vi "GUI.DisableState.Set.vi"(7 "Enable?":bool=TRUE, 8 "error in (no error)":errorcluster, 11 "State Variables in":T1) -> (0 "error out":errorcluster, 3 "State Variables out":T1)   [LabVIEW 2025, in "XNET Bus Monitor Client.lvlib"]
uses:
  XNET Bus Monitor Client.lvlib
  Types/GUI.StateVariables.ctl
  Types/StreamEngine.CmdQueueData.ctl
  Types/StreamEngine.CmdQueueData.Cmd.ctl
  Types/StreamEngine.QueueRefs.ctl
  Types/GUI.Controls.Refs.ctl
  <vilib>/gRPC/LabVIEW gRPC Library/Shared/grpcId.ctl
  <vilib>/gRPC/LabVIEW gRPC Library/grpc-lvsupport-release.lvlib
  xnet_can_bus_monitor_api_client/RPC Messages/ni_xnet_can_bm_api_DirectionFilter.ctl
  xnet_can_bus_monitor_api_client/xnet_can_bus_monitor_api_client.lvlib
  xnet_can_bus_monitor_api_client/RPC Messages/ni_xnet_can_bm_api_FrameFilter.ctl
  Types/gRPC.ConnectionInfo.ctl
  Types/SubProcessEngine.CmdQueueData.ctl
  Types/SubProcessEngine.CmdQueueData.Cmd.ctl
  Types/SubProcessEngine.QueueRefs.ctl
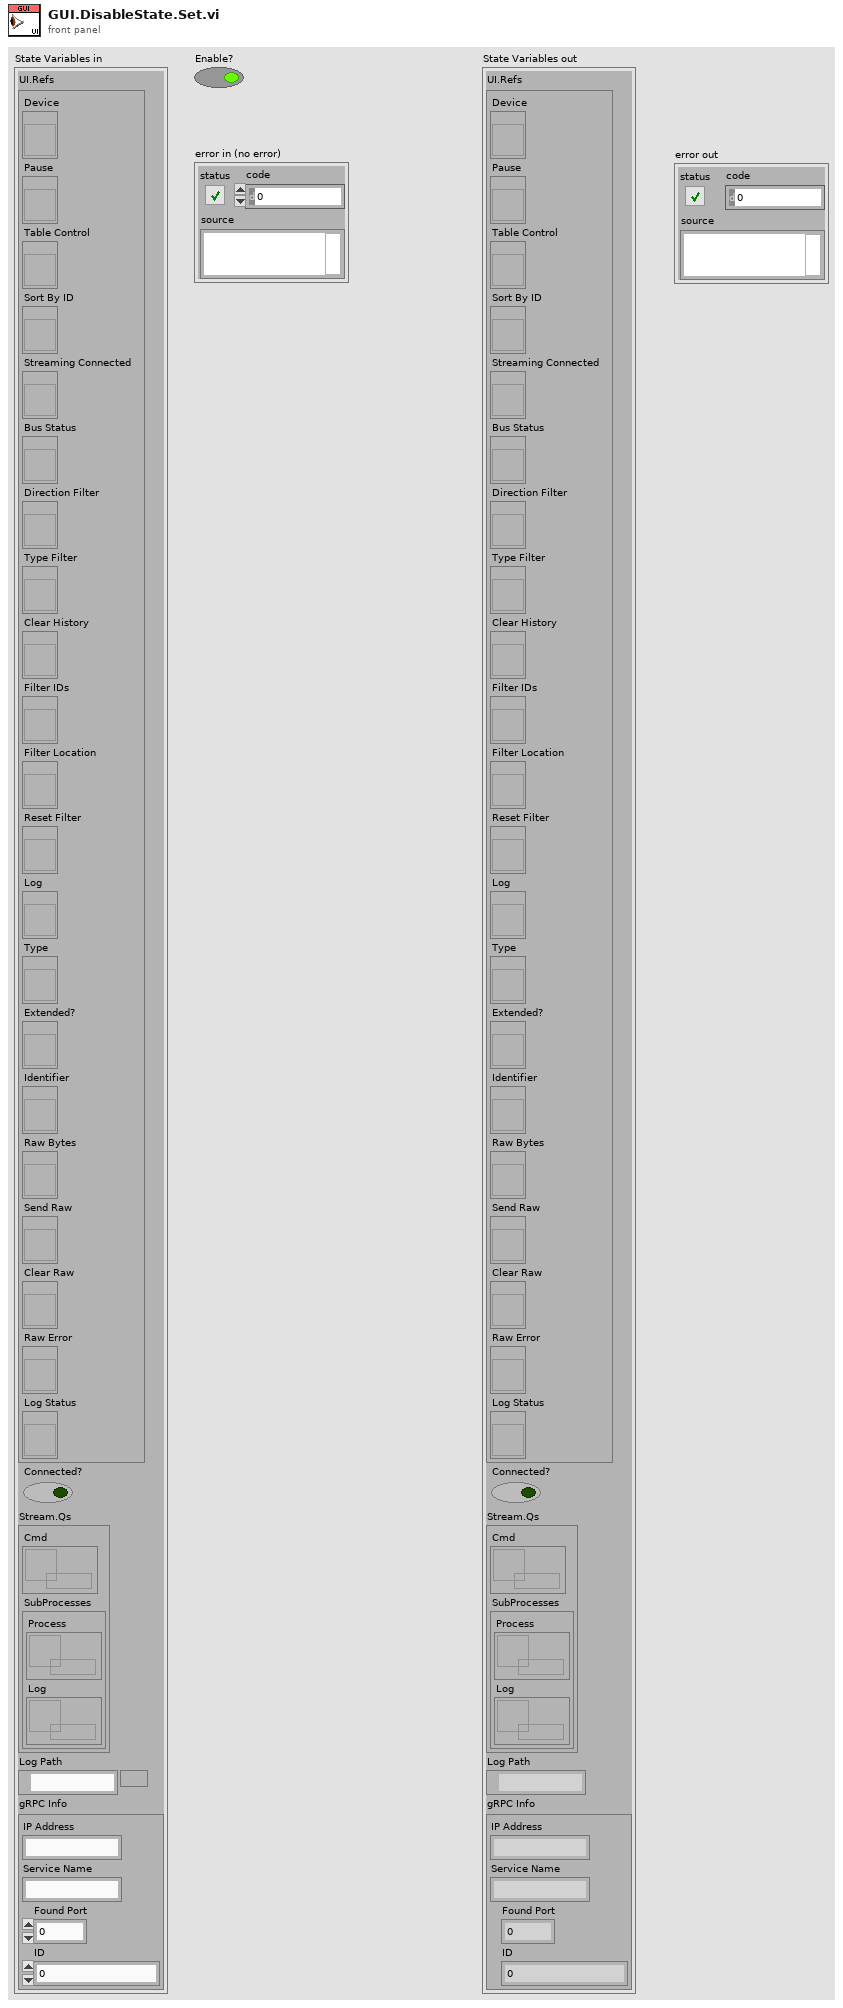
[diagram p1: front panel]
types:
  T1 = typedef "XNET Bus Monitor Client.lvlib/GUI.StateVariables.ctl" = cluster{"UI.Refs":T2, "Connected?":bool, "Stream.Qs":T3, "Log Path":path, "gRPC Info":T5}
  T2 = typedef "XNET Bus Monitor Client.lvlib/GUI.Controls.Refs.ctl" = cluster{"Device":refnum<vi>, "Pause":refnum<vi>, "Table Control":refnum<vi>, "Sort By ID":refnum<vi>, "Streaming Connected":refnum<vi>, "Bus Status":refnum<vi>, "Direction Filter":refnum<vi>, "Type Filter":refnum<vi>, "Clear History":refnum<vi>, "Filter IDs":refnum<vi>, "Filter Location":refnum<vi>, "Reset Filter":refnum<vi>, "Log":refnum<vi>, "Type":refnum<vi>, "Extended?":refnum<vi>, "Identifier":refnum<vi>, "Raw Bytes":refnum<vi>, "Send Raw":refnum<vi>, "Clear Raw":refnum<vi>, "Raw Error":refnum<vi>, "Log Status":refnum<vi>}
  T3 = typedef "XNET Bus Monitor Client.lvlib/StreamEngine.QueueRefs.ctl" = cluster{"Cmd":refnum<queue>, "SubProcesses":T4}
  T4 = typedef "XNET Bus Monitor Client.lvlib/SubProcessEngine.QueueRefs.ctl" = cluster{"Process":refnum<queue>, "Log":refnum<queue>}
  T5 = typedef "XNET Bus Monitor Client.lvlib/gRPC.ConnectionInfo.ctl" = cluster{"IP Address":string, "Service Name":string, "Found Port":u64, "ID":T6}
  T6 = typedef "grpc-lvsupport-release.lvlib/grpcId.ctl" = u64
  T7 = enum8{"Enabled", "Disabled", "Disabled and Grayed Out"}
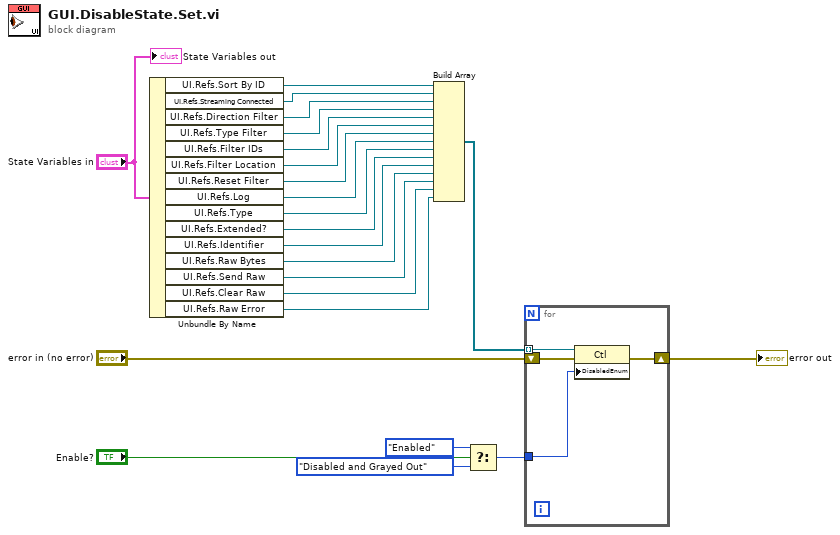
[diagram p0: block diagram]
diagram:
  n1 = Unbundle By Name("State Variables in") -> ("UI.Refs.Sort By ID"=w16:refnum<vi>, "UI.Refs.Streaming Connected"=w15:refnum<vi>, "UI.Refs.Direction Filter"=w14:refnum<vi>, "UI.Refs.Type Filter"=w13:refnum<vi>, "UI.Refs.Filter IDs"=w12:refnum<vi>, "UI.Refs.Filter Location"=w11:refnum<vi>, "UI.Refs.Reset Filter"=w10:refnum<vi>, "UI.Refs.Log"=w9:refnum<vi>, "UI.Refs.Type"=w7:refnum<vi>, "UI.Refs.Extended?"=w6:refnum<vi>, "UI.Refs.Identifier"=w5:refnum<vi>, "UI.Refs.Raw Bytes"=w4:refnum<vi>, "UI.Refs.Send Raw"=w3:refnum<vi>, "UI.Refs.Clear Raw"=w2:refnum<vi>, "UI.Refs.Raw Error"=w1:refnum<vi>)
  n2 = Build Array(w16, w15, w14, w13, w12, w11, w10, w9, w7, w6, w5, w4, w3, w2, w1) -> (w8:refnum<vi>[])
  n3 = Select(t=T7."Enabled" ("Disabled"), s="Enable?", f=T7."Disabled and Grayed Out" ("Disabled")) -> (s? t:f=w18:T7)
  n4 = for {
    shift-right: [w26] -> w23
    shift-left: "error in (no error)" -> [w27]
    tunnel: w18 -> [w25]
    tunnel: w8 -> [w24] mode=indexing
    n5 = property class="Ctl"(reference=w24, error in=w27, "DisabledEnum"=w25) -> (error out=w26:errorcluster)  [unwired: 1 out]
  }
  "error out" <- w23
  "State Variables out" <- "State Variables in"
